vi "Get Thread UI.vi"(8 "error in (no error)":errorcluster, 11 "Component UI in":refnum<class "UDPlog User Interfaces.lvclass">) -> (0 "error out":errorcluster, 2 "Thread Settings UI":refnum<class "User Interface.lvclass">, 3 "Component UI out":refnum<class "UDPlog User Interfaces.lvclass">)   [LabVIEW 2023, in "UDPlog.lvlib" / "UDPlog User Interfaces.lvclass"]
uses:
  UDPlog User Interfaces.lvclass
  Users/Public/Documents/National Instruments/NI VeriStand 2023/Custom Devices/Data Sharing Framework/Linux_x64/DSF Core.lvlibp/Classes/User Interface/User Interface.lvclass
  Thread/UDPlog Thread User Interface.lvclass
  C:/Users/Public/Documents/National Instruments/NI VeriStand 2023/Custom Devices/Data Sharing Framework/Linux_x64/DSF Core.lvlibp/Classes/User Interface/User Interface.lvclass
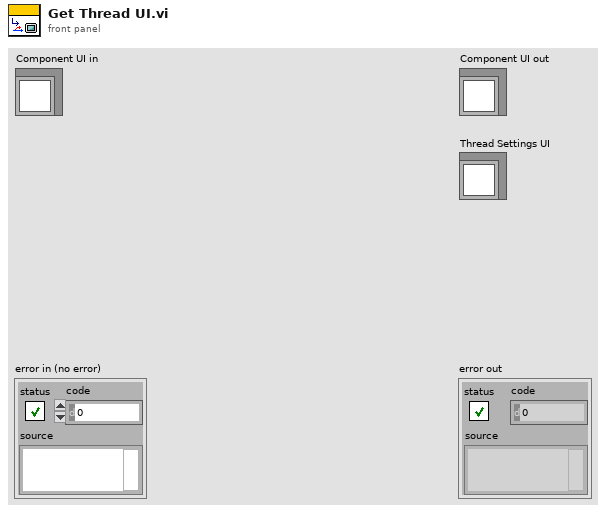
[diagram p1: front panel]
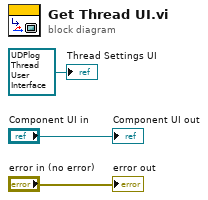
[diagram p0: block diagram]
diagram:
  "error out" <- "error in (no error)"
  "Component UI out" <- "Component UI in"
  "Thread Settings UI" <- refnum<class "UDPlog Thread User Interface.lvclass"> refnum ("UDPlog.lvlib:UDPlog Thread User Interface.lvclass")
